vi "Create_AO_POLAR_WF.vi"(8 "error in":errorcluster) -> (0 "error out":errorcluster)   [LabVIEW 2025]
uses:
  <vilib>/Waveform/WDTOps.llb/WDT Append Waveforms DBL.vi
panel:
  out "Illumination analog waveforms":waveform(dbl)(graph) caption="Output Waveform"
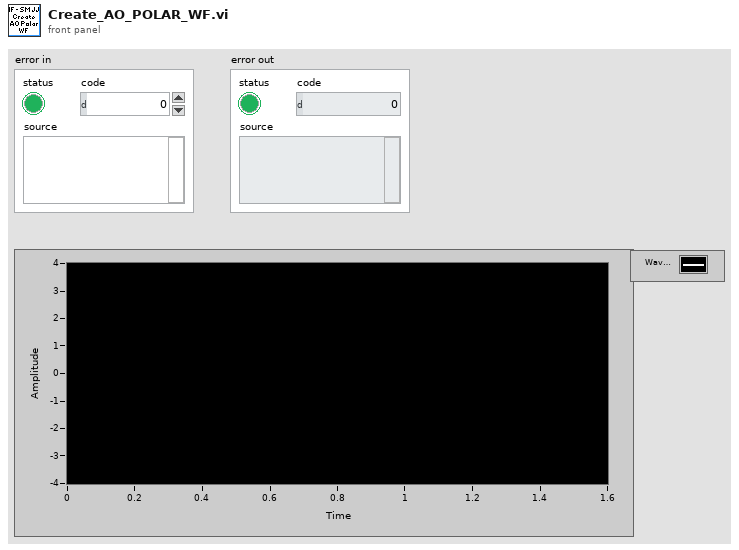
[diagram p1: front panel]
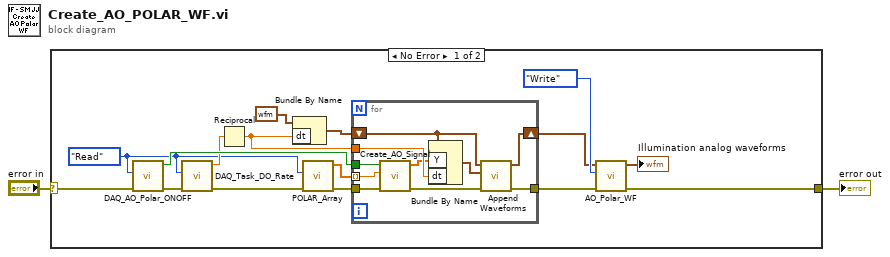
[diagram p0: block diagram]
diagram:
  n1 = case shown="No Error" "error in" {
    selector: "error in" -> [w18 w29]
    tunnel: [w17 w29] -> w1
    frame No Error {
      w12 = enum16{"Write", "Read"}."Read" ("Action")
      n2 = call "DAQ_AO_Polar_ONOFF.vi"("error in"=w18, "Action"=w12) -> ("error out"=w14:errorcluster, "ON / OFF"=w15:bool)  [unwired: 8 in]
      n3 = call "DAQ_Task_DO_Rate.vi"("error in"=w14, "Action"=w12) -> ("error out"=w11:errorcluster, "DO_Rate"=w13:dbl)  [unwired: 8 in]
      n4 = Reciprocal(x=w13) -> (1/x=w6:dbl)
      n5 = Bundle By Name(cluster=waveform(dbl) {"t0"=timestamp(0 s since 1904-01-01), "dt"=0.001, "Y"=[]} ("waveform out"), "dt"=w6) -> (w5:waveform(dbl))
      n6 = call "POLAR_Array.vi"("error in"=w11, "Action"=w12) -> ("error out"=w9:errorcluster, "Pockels_Array"=w10:dbl[])  [unwired: 8 in]
      n7 = for {
        tunnel: [w21] -> w3
        tunnel: w15 -> [w28]
        tunnel: w6 -> [w27]
        tunnel: w10 -> [w25] mode=indexing
        tunnel: w9 -> [w24]
        shift-right: [w22] -> w4
        shift-left: w5 -> [w19]
        n8 = call "Create_AO_Signal.vi"("error in"=w24, "AO Amplitude"=w25, "ON / OFF"=w28) -> ("error out"=w23:errorcluster, "WF"=w26:dbl[])  [unwired: 7 in]
        n9 = Bundle By Name(cluster=w19, "Y"=w26, "dt"=w27) -> (w20:waveform(dbl))
        n10 = call-poly <vilib>:"Append Waveforms.vi"("error in (no error)"=w23, "waveform B"=w20, "waveform A"=w19) -> ("error out"=w21:errorcluster, "waveform out"=w22:waveform(dbl))  [unwired: 7 in]
      }
      n11 = call "AO_Polar_WF.vi"("error in"=w3, "Action"=enum16{"Write", "Read"}."Write", "AO Polar WF"=w4) -> ("error out"=w17:errorcluster, "AO Poalr WF"=→"Illumination analog waveforms":waveform(dbl))  [unwired: 7 in]
    }
    frame Error {
    }
  }
  "error out" <- w1
